vi "Excel Find and Replace (num).vi"(0 "report in":refnum<class "NI_report.lvclass">, 5 "searched string":string, 7 "replacement":dbl format="%.2f", 9 "format string (%.3f)":string, 11 "error in (no error)":errorcluster) -> (4 "report out":refnum<class "NI_report.lvclass">, 8 "found?":bool, 15 "error out":errorcluster)   [LabVIEW 2016, in "NI_Excel.lvclass"]
doc: "Searches the occurrences of <B>searched string</B> and replaces them with a new string or numeric value. The data type you wire to the <B>replacement</B> input determines the polymorphic instance to use."
uses:
  <vilib>/Utility/NIReport.llb/Excel/NI_Excel.lvclass
  <vilib>/Utility/NIReport.llb/NI_report.lvclass
  C:/Program Files (x86)/National Instruments/LabVIEW 2016/vi.lib/Utility/NIReport.llb/NI_report.lvclass
  <vilib>/Utility/NIReport.llb/Excel/NI_Excel.lvclass/NI_Excel.ctl
  <vilib>/Utility/NIReport.llb/NI_ReportGenerationCore.lvlib
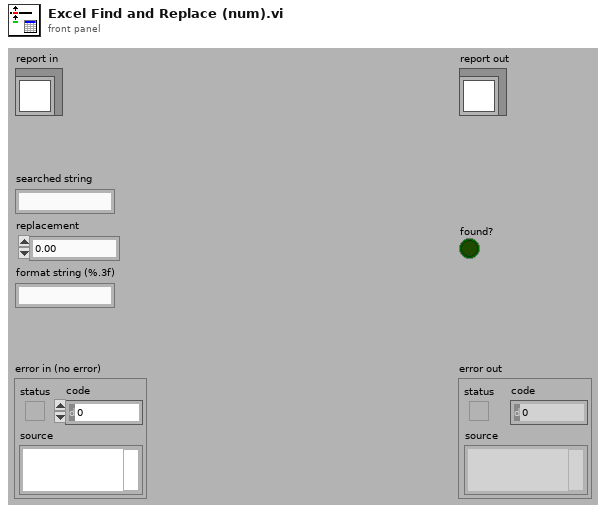
[diagram p1: front panel]
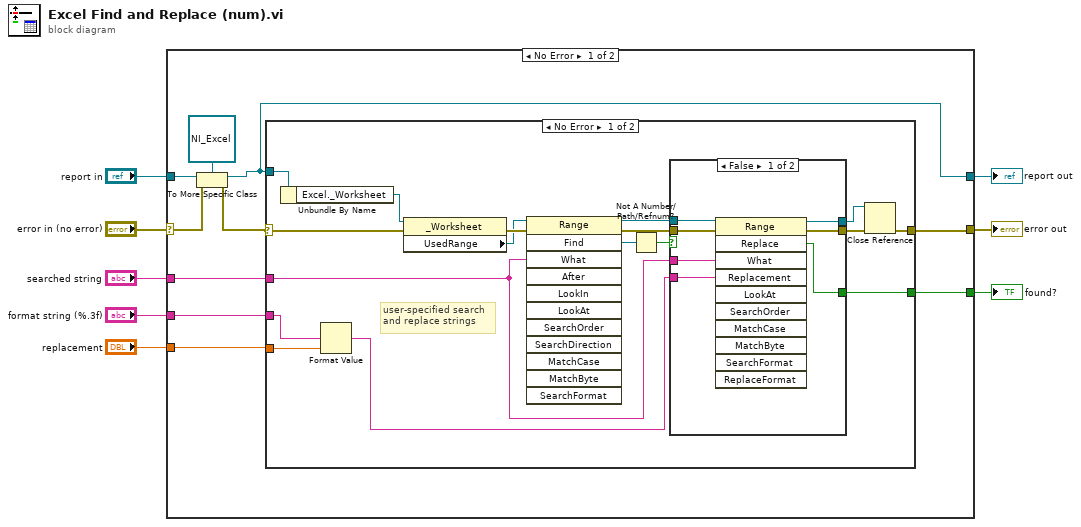
[diagram p0: block diagram]
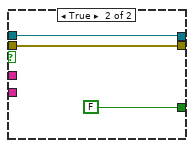
[diagram p2: hidden frame]
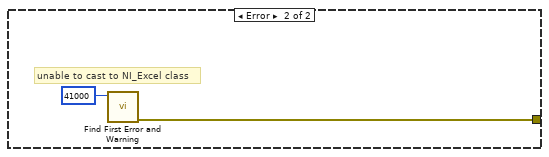
[diagram p3: hidden frame]
diagram:
  n1 = case shown="No Error" "error in (no error)" {
    selector: "error in (no error)" -> [w16 w49]
    tunnel: [w10 w49] -> w7
    tunnel: [w15 w48] -> w5
    tunnel: "report in" -> [w17 w48]
    tunnel: "format string (%.3f)" -> [w12 _]
    tunnel: "replacement" -> [w11 _]
    tunnel: "searched string" -> [w13 _]
    tunnel: [w9 _] -> w1
    frame No Error {
      n2 = To More Specific Class(target class=refnum<class "NI_Excel.lvclass"> refnum ("report in"), reference=w17, error in=w16) -> (specific class reference=w15:refnum<class "NI_Excel.lvclass">, error out=w14:errorcluster)
      n3 = case shown="No Error" w14 {
        selector: w14 -> [w33 _]
        tunnel: [w34 w46] -> w10
        tunnel: [w24 _] -> w9
        tunnel: w15 -> [w23 _]
        tunnel: w13 -> [w19 _]
        tunnel: w12 -> [w22 _]
        tunnel: w11 -> [w21 _]
        frame No Error {
          # "user-specified search\nand replace strings"
          n4 = Unbundle By Name(w23) -> ("Excel._Worksheet"=w35:refnum<k7>)
          n5 = Format Value(format string=w22, value (0)=w21) -> (output string=w20:string)  [unwired: 1 out]
          n6 = property class="_Worksheet"(reference=w35, error in=w33) -> (error out=w32:errorcluster, "UsedRange"=w31:refnum<k7>)  [unwired: 1 out]
          n7 = invoke class="Range" method="Find"(reference=w31, error in=w32, "What"=w19) -> (reference out=w28:refnum<k7>, error out=w27:errorcluster, "Find"=w30:refnum<k7>)  [unwired: 9 in, 9 out]
          n8 = Not A Number/Path/Refnum?(number/path/refnum=w30) -> (NaN/Path/Refnum?=w29:bool)
          n9 = case shown="False" w29 {
            tunnel: w19 -> [w42 _]
            tunnel: w20 -> [w41 _]
            tunnel: w28 -> [w40 w45]
            tunnel: [w39 w45] -> w25
            tunnel: w27 -> [w38 w44]
            tunnel: [w37 w44] -> w26
            tunnel: [w36 FALSE ("found?")] -> w24
            frame False {
              n10 = invoke class="Range" method="Replace"(reference=w40, error in=w38, "What"=w42, "Replacement"=w41) -> (reference out=w39:refnum<k7>, error out=w37:errorcluster, "Replace"=w36:bool)  [unwired: 7 in, 8 out]
            }
            frame True {
            }
          }
          n11 = Close Reference(reference=w25, error in (no error)=w26) -> (error out=w34:errorcluster)
        }
        frame Error {
          # "unable to cast to NI_Excel class"
          n12 = call <vilib>:"Find First Error and Warning.vi"("error code"=41000) -> ("error out"=w46:errorcluster)  [unwired: 2 in, 4 out]
        }
      }
    }
    frame Error {
    }
  }
  "error out" <- w7
  "report out" <- w5
  "found?" <- w1
